vi "Fetch Measurement.vi"   [LabVIEW 2020, in "Agilent B2900 Series.lvlib"]
doc: "Return the measurement data\n\n<B>Note:</B> Use this VI only with other low-level VIs. The high-level VIs automatically incorporate this functionality. This VI does not check the instrument status."
uses:
  Agilent B2900 Series.lvlib
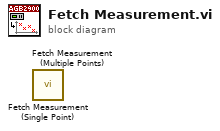
[diagram p0: block diagram]
diagram:
  n1 = call "Fetch Measurement (Single Point).vi"() -> ()  [unwired: 9 in, 3 out]
  n2 = call "Fetch Measurement (Multiple Points).vi"() -> ()  [unwired: 9 in, 3 out]
